vi "PutGetTreeNodeExample.vi"() -> ()   [LabVIEW 2015]
uses:
  Library/MDSplus.lvlib
panel:
  out "Time inserted":string="my_tree"
  in  "Path":string=":NUM0"
  in  "Tree Shot":i32=-1
  in  "Tree Name":string="my_tree"
  in  "Value In":sgl=5.555
  out "Value Out":sgl
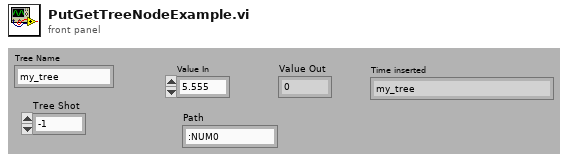
[diagram p1: front panel]
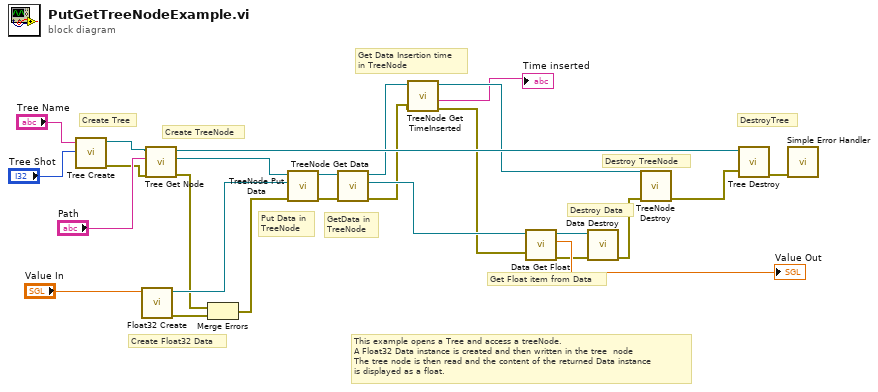
[diagram p0: block diagram]
diagram:
  # "Get Data Insertion time\nin TreeNode"
  # "This example opens a Tree and access a treeNode.\nA Float32 Data instance is created and then written in the tree  node\nThe tree node is then read and the content of the returned Data instance\nis displayed as a float."
  # "DestroyTree"
  # "Destroy TreeNode"
  # "Destroy Data"
  # "Get Float item from Data"
  # "GetData in\nTreeNode"
  # "Put Data in\nTreeNode"
  # "Create Float32 Data"
  # "Create TreeNode"
  # "Create Tree"
  n1 = call "Tree Create.vi"("Shot"="Tree Shot", "Name"="Tree Name") -> ("error out"=w9:errorcluster, "Tree DVR out"=w8:refnum<data-value>)  [unwired: 8 in]
  n2 = call "Float32 Create.vi"("SGL in"="Value In") -> ("error out"=w22:errorcluster, "Float32 DVR out"=w24:refnum<data-value>)  [unwired: 9 in]
  n3 = call "Tree Get Node.vi"("error in (no error)"=w9, "Path"="Path", "Tree DVR in"=w8) -> ("error out"=w13:errorcluster, "Node out"=w14:refnum<data-value>, "Tree DVR out"=w7:refnum<data-value>)  [unwired: 6 in]
  n4 = Merge Errors(w13, w22) -> (w23:errorcluster)
  n5 = call "TreeNode Put Data.vi"("error in (no error)"=w23, "Data"=w24, "TreeNode DVR in"=w14) -> ("error out"=w20:errorcluster, "TreeNode DVR out"=w21:refnum<data-value>)  [unwired: 7 in]
  n6 = call "TreeNode Get Data.vi"("error in (no error)"=w20, "TreeNode DVR in"=w21) -> ("error out"=w3:errorcluster, "Data out"=w6:refnum<data-value>, "TreeNode DVR out"=w5:refnum<data-value>)  [unwired: 7 in]
  n7 = call "TreeNode Get TimeInserted.vi"("error in (no error)"=w3, "TreeNode DVR in"=w5) -> ("error out"=w2:errorcluster, "TimeInserted String out"=→"Time inserted":string, "TreeNode DVR out"=w4:refnum<data-value>)  [unwired: 6 in, 1 out]
  n8 = call "Data Get Float.vi"("error in (no error)"=w2, "Data DVR in"=w6) -> ("error out"=w17:errorcluster, "SGL out"=→"Value Out":sgl, "Data DVR out"=w19:refnum<data-value>)  [unwired: 7 in]
  n9 = call "Data Destroy.vi"("error in (no error)"=w17, "Data DVR in"=w19) -> ("error out"=w16:errorcluster)  [unwired: 9 in]
  n10 = call "TreeNode Destroy.vi"("error in (no error)"=w16, "TreeNode DVR in"=w4) -> ("error out"=w12:errorcluster)  [unwired: 9 in]
  n11 = call "Tree Destroy.vi"("error in (no error)"=w12, "Tree DVR in"=w7) -> ("error out"=w15:errorcluster)  [unwired: 9 in]
  n12 = call <vilib>:"Simple Error Handler.vi"("error in (no error)"=w15) -> ()  [unwired: 4 in, 5 out]
